vi "TWM Client Compare Version Strings.vi"(1 "version b":string, 2 "version a":string) -> (0 "a>b, a=b, a<b {+1,0,-1}":i32)   [LabVIEW 2020, in "TWM Client.lvlib"]
doc: "Comparator of version strings."
uses:
  TWM Client.lvlib
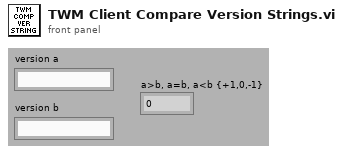
[diagram p1: front panel]
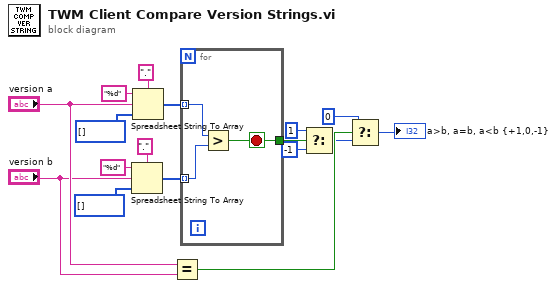
[diagram p0: block diagram]
diagram:
  n1 = Spreadsheet String To Array(delimiter (Tab)=".", format string="%d", spreadsheet string="version b", array type (2D Dbl)=i32[] []) -> (array=w10:i32[])
  n2 = Spreadsheet String To Array(delimiter (Tab)=".", format string="%d", spreadsheet string="version a", array type (2D Dbl)=i32[] []) -> (array=w11:i32[])
  n3 = Equal?(x="version a", y="version b") -> (x = y?=w7:bool)
  n4 = for {
    tunnel: w11 -> [w18] mode=indexing
    tunnel: w10 -> [w20] mode=indexing
    tunnel: [w19] -> w6
    stop <- w19 stop-if-true
    n5 = Greater?(x=w18, y=w20) -> (0:w19:bool)
  }
  n6 = Select(t=1, s=w6, f=-1) -> (s? t:f=w3:i32)
  n7 = Select(t=0, s=w7, f=w3) -> (s? t:f=→"a>b, a=b, a<b {+1,0,-1}":i32)
